vi "Test-coil.vi"() -> ()   [LabVIEW 2020, in "PowerControl.lvlib"]
uses:
  YP03-60_X/YP03-60_X.lvclass
  YP03-60_Y/YP03-60_Y.lvclass
  YP03-60_Z/YP03-60_Z.lvclass
  PowerControl.lvlib
panel:
  in  "Output((F) Z":bool
  in  "Output((F) X":bool
  in  "OutputY((F)":bool
  in  "Current(0) Y":dbl
  in  "Current(0) X":dbl
  in  "Current(0) Z":dbl
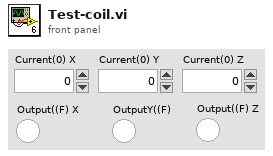
[diagram p1: front panel]
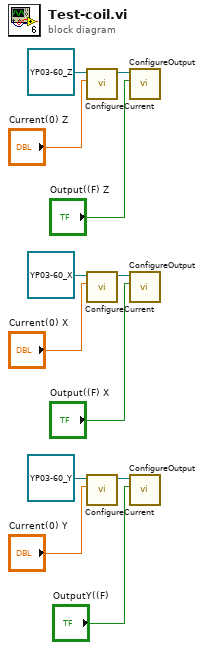
[diagram p0: block diagram]
diagram:
  n1 = call-dynamic "ConfigureCurrent.vi"("Current(0)"="Current(0) Z", "YP03-60_Z in"=refnum<class "YP03-60_Z.lvclass"> refnum ("PowerControl.lvlib:YP03-60_Z.lvclass")) -> ("YP03-60_Z out"=w1:refnum<class "YP03-60_Z.lvclass">)  [unwired: 8 in, 1 out]
  n2 = call-dynamic "ConfigureCurrent.vi"("Current(0)"="Current(0) X", "YP03-60_X in"=refnum<class "YP03-60_X.lvclass"> refnum ("PowerControl.lvlib:YP03-60_X.lvclass")) -> ("YP03-60_X out"=w8:refnum<class "YP03-60_X.lvclass">)  [unwired: 8 in, 1 out]
  n3 = call-dynamic "ConfigureCurrent.vi"("Current(0)"="Current(0) Y", "YP03-60_Y in"=refnum<class "YP03-60_Y.lvclass"> refnum ("PowerControl.lvlib:YP03-60_Y.lvclass")) -> ("YP03-60_Y out"=w9:refnum<class "YP03-60_Y.lvclass">)  [unwired: 8 in, 1 out]
  n4 = call-dynamic "ConfigureOutput.vi"("Output((F)"="Output((F) Z", "YP03-60_Z in"=w1) -> ()  [unwired: 8 in, 2 out]
  n5 = call-dynamic "ConfigureOutput.vi"("Output((F)"="Output((F) X", "YP03-60_X in"=w8) -> ()  [unwired: 8 in, 2 out]
  n6 = call-dynamic "ConfigureOutput.vi"("Output((F)"="OutputY((F)", "YP03-60_Y in"=w9) -> ()  [unwired: 8 in, 2 out]
